vi "Read Counter.vi"(8 "error in (no error)":errorcluster, 11 "SD Module in":refnum<class "SD Module.lvclass">) -> (0 "error out":errorcluster, 2 "Counter":T1 {"Counter Channels"."Frequency Measurement"."Measurement Timebase" items=["256 us", "512 us", "1024 us", "2048 us", "4096 us", "8192 us", "16384 us", "32768 us"]; "Counter Channels"."Frequency Measurement"."Measurement Edge" items=["Rising Edge", "Falling Edge"]; "Counter Channels"."Pulse Width Measurement"."Measurement Type" items=["High Pulse"=3, "Low Pulse"=4, "Most Recent"=5]; "Counter Channels"."Period Measurement"."Measurement Edge" items=["Rising Edge", "Falling Edge"]; "Counter Channels"."Count Edges"."Gate Mode" items=["Next Channel"=1, "Always Enabled"=3]; "Counter Channels"."Count Edges"."Output Mode" items=["Toggle, Reset Off", "Toggle, Reset On", "On Pulse", "Off Pulse"]; "Counter Channels"."Count Edges"."Counter Direction" items=["Count up", "Count down"]; "Counter Channels"."Count Edges"."Counter Source" items=["This Channel", "Terminal count of previous channel"]; "Counter Channels"."Count Edges"."Counter Event" items=["Rising Edge", "Falling Edge", "Any Edge"]; "Counter Channels"."Measurement Mode" items=["Count Edges", "Period Measurements", "Pulse Width Measurements", "Frequency Measurements"]}, 3 "SD Module out":refnum<class "SD Module.lvclass">)   [LabVIEW 2020, in "Modules.lvlib" / "SD Module.lvclass"]
uses:
  SD Module.lvclass
  Type Defs/Counter.ctl
  Type Defs/Counter Channel.ctl
  Type Defs/Count Edges.ctl
  Type Defs/Period Measurement.ctl
  Type Defs/Pulse Width Measurement.ctl
  Type Defs/Frequency Measurement.ctl
  SD Module.lvclass/SD Module.ctl
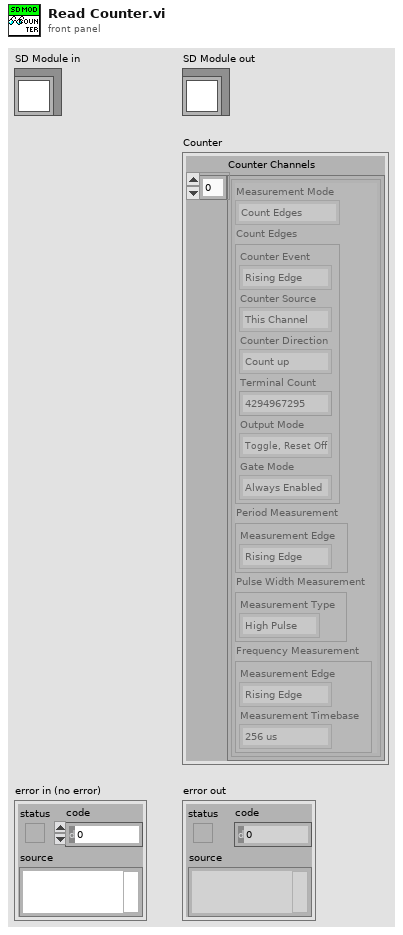
[diagram p1: front panel]
types:
  T1 = typedef "Modules.lvlib/SD Module.lvclass/Counter.ctl" = cluster{"Counter Channels":T2[]}
  T2 = typedef "Modules.lvlib/SD Module.lvclass/Counter Channel.ctl" = cluster{"Measurement Mode":u32, "Count Edges":T3, "Period Measurement":T4, "Pulse Width Measurement":T5, "Frequency Measurement":T6}
  T3 = typedef "Modules.lvlib/SD Module.lvclass/Count Edges.ctl" = cluster{"Counter Event":u32, "Counter Source":u32, "Counter Direction":u32, "Terminal Count":u32, "Output Mode":u32, "Gate Mode":u32}
  T4 = typedef "Modules.lvlib/SD Module.lvclass/Period Measurement.ctl" = cluster{"Measurement Edge":u32}
  T5 = typedef "Modules.lvlib/SD Module.lvclass/Pulse Width Measurement.ctl" = cluster{"Measurement Type":u32}
  T6 = typedef "Modules.lvlib/SD Module.lvclass/Frequency Measurement.ctl" = cluster{"Measurement Edge":u32, "Measurement Timebase":u32}
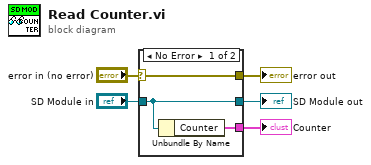
[diagram p0: block diagram]
diagram:
  n1 = case shown="No Error" "error in (no error)" {
    selector: "error in (no error)" -> [w8 w9]
    tunnel: [w8 w9] -> w4
    tunnel: [w7 w10] -> w2
    tunnel: "SD Module in" -> [w7 w10]
    tunnel: [w6 _] -> w1
    frame No Error {
      n2 = Unbundle By Name(w7) -> ("Counter"=w6:T1)
    }
    frame Error {
    }
  }
  "error out" <- w4
  "SD Module out" <- w2
  "Counter" <- w1
